vi "IntensityCubetoRGBScale.vi"(1 "Router":u32, 2 "Plane":u32, 3 "Trace":u32[][][][](array[numeric]), 4 "threshold":cluster{"max":u32, "min":u32}) -> (0 "RGB Scale":u32[][](array[numeric]))   [LabVIEW 2009]
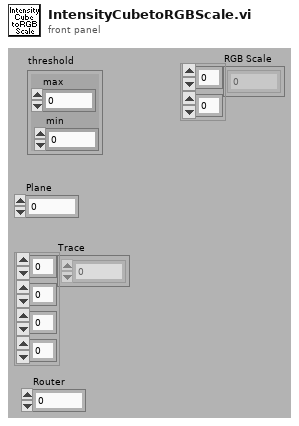
[diagram p1: front panel]
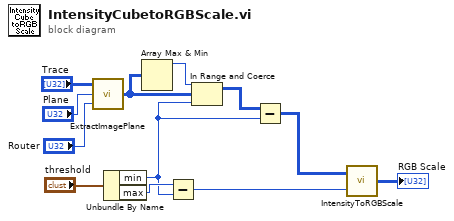
[diagram p0: block diagram]
diagram:
  n1 = call "ExtractImagePlane.vi"("Router"="Router", "Plane"="Plane", "Trace"="Trace") -> ("Intensity"=w5:u32[][])
  n2 = Unbundle By Name("threshold") -> ("min"=w2:u32, "max"=w6:u32)
  n3 = Array Max & Min(array=w5) -> (max value=w4:u32)  [unwired: 3 out]
  n4 = Subtract(x=w6, y=w2) -> (x-y=w7:u32)
  n5 = In Range and Coerce(upper limit=w4, x=w5, lower limit=w2) -> (coerced(x)=w3:u32[][])  [unwired: 1 out]
  n6 = Subtract(x=w3, y=w2) -> (x-y=w1:u32[][])
  n7 = call "IntensityToRGBScale.vi"("Threshold (max)"=w7, "Intensity"=w1) -> ("RGB Scale"=→"RGB Scale":u32[][])
